vi "CancelTimeoutNotifier.vi"(8 "error in (no error)":errorcluster, 11 "Lockin Error Timeout":refnum<notifier>) -> (0 "error out":errorcluster)   [LabVIEW 2019, in "AFM_Litho_Plugin.IV.lvclass"]
uses:
  AFM_Litho_Plugin.IV.lvclass
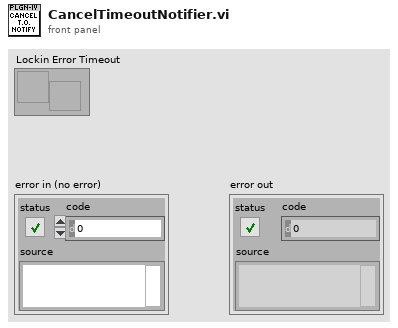
[diagram p1: front panel]
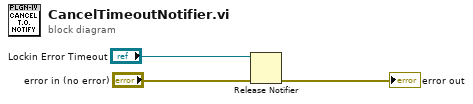
[diagram p0: block diagram]
diagram:
  n1 = Release Notifier(notifier="Lockin Error Timeout", error in (no error)="error in (no error)") -> (error out=→"error out":errorcluster)  [unwired: 1 in, 2 out]
